vi "clickpoints.vi"(8 "Err_In":errorcluster) -> (0 "error out":errorcluster caption="Err_Out", 2 "MouseMoves":cdb[](array[numeric]), 3 "Points":cdb[](array[numeric]))   [LabVIEW 2012]
doc: "This VI can be used for interactive point definition. If you click with the left mouse key, the purrent position of the mouse (in screen coordinates) is added to an array.\nIf you click with another mouse button, the interactive point definition will be finished.\n\nThe VI works almost like \"mausi.vi\". The difference here: The VI will be finished by a click with the middle or right mouse key."
uses:
  <vilib>/Utility/inputDevices.llb/mouseAcquire.vi
  <vilib>/Utility/inputDevices.llb/closeMouse.vi
panel:
  out "NoOfPTS":i32
  out "Movement":bool
  out "XY-Graph":cluster{dbl[], dbl[]}[](graph)
  out "button info":T1 caption="KeyInfo"
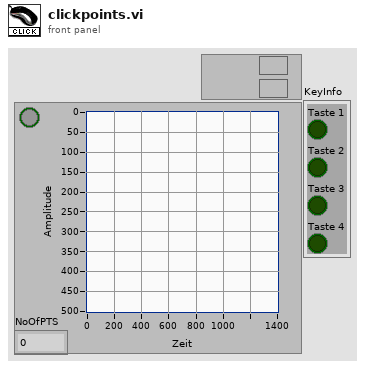
[diagram p1: front panel]
types:
  T1 = cluster{"button 1":bool, "button 2":bool, "button 3":bool, "button 4":bool}
  T2 = cluster{"Horizontal":i32, "Vertical":i32, "Scrolling":i32}
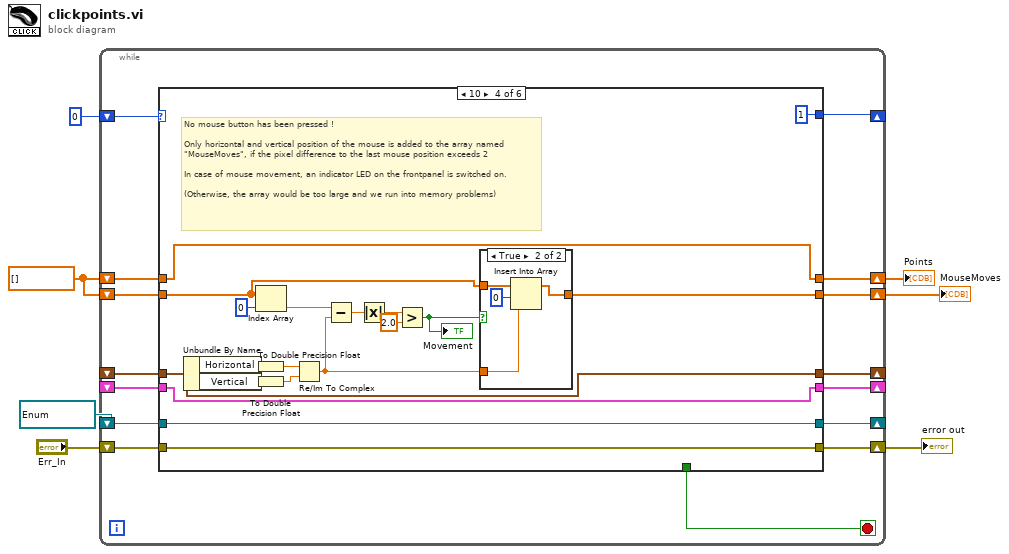
[diagram p0: block diagram]
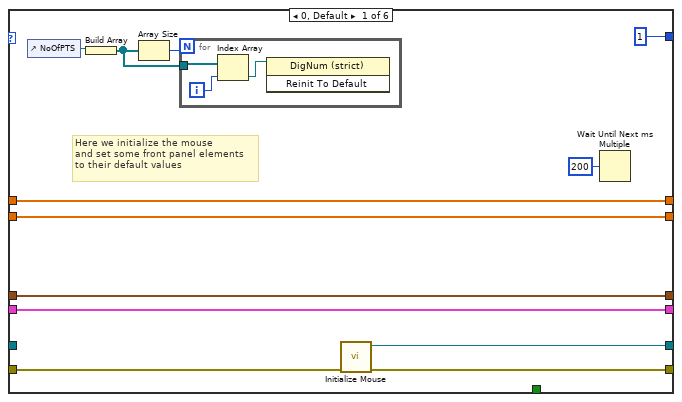
[diagram p2: hidden frame]
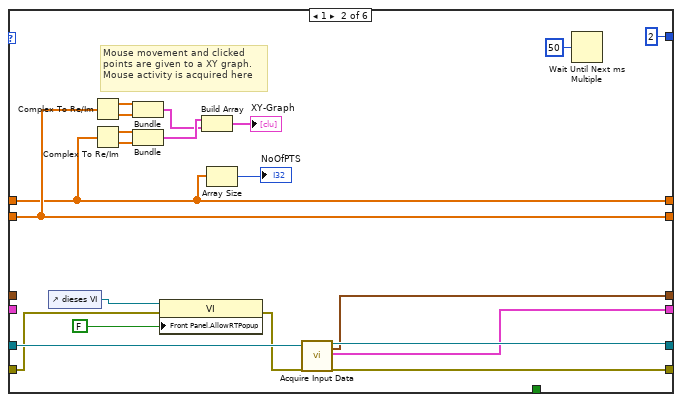
[diagram p3: hidden frame]
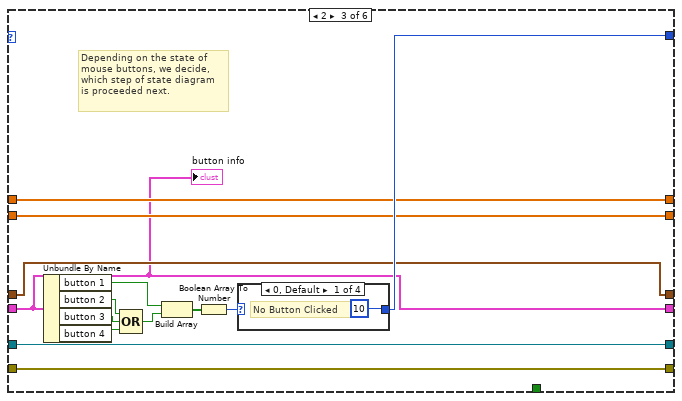
[diagram p4: hidden frame]
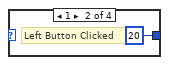
[diagram p5: hidden frame]
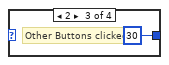
[diagram p6: hidden frame]
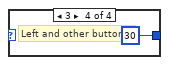
[diagram p7: hidden frame]
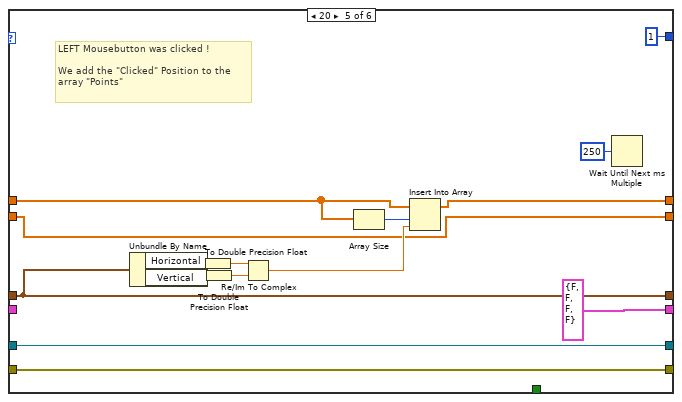
[diagram p9: hidden frame]
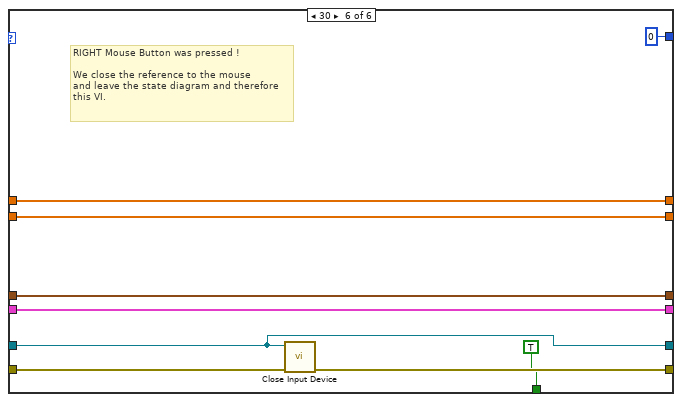
[diagram p10: hidden frame]
diagram:
  w1 = cdb[] []
  w4 = refnum<k1> refnum items=["MOUSE"] ("device ID")
  n1 = while {
    shift-right: [w20] -> w5
    shift-left: "Err_In" -> [w21]
    shift-right: [w19] -> _
    shift-left: w4 -> [w17]
    shift-right: [w18] -> _
    shift-left: 0 ("Numerisches Element") -> [w22]
    shift-right: [w16] -> _
    shift-left: _ -> [w13]
    shift-right: [w15] -> _
    shift-left: _ -> [w14]
    shift-right: [w12] -> w2
    shift-left: w1 -> [w11]
    shift-right: [w10] -> w3
    shift-left: w1 -> [w9]
    stop <- w8 stop-if-true
    n2 = case shown="10" w22 {
      tunnel: w21 -> [w34 w40 w60 w88 w104 w124]
      tunnel: [w33 w58 w60 w88 w104 w123] -> w20
      tunnel: [w32 w56 w61 w87 w105 w116] -> w19
      tunnel: [1 ("Numerisches Element") 2 ("Numerisches Element") w65 1 ("Numerisches Element") 1 ("Numerisches Element") 0 ("Numerisches Element")] -> w18
      tunnel: w17 -> [_ w57 w61 w87 w105 w116]
      tunnel: [w29 w54 w62 w85 w106 w121] -> w16
      tunnel: [w30 w53 w59 w86 T1 {"button 1"=FALSE, "button 2"=FALSE, "button 3"=FALSE, "button 4"=FALSE} ("button info") w122] -> w15
      tunnel: w14 -> [w30 _ w59 w86 _ w122]
      tunnel: w13 -> [w29 _ w62 w85 w106 w121]
      tunnel: [w27 w47 w64 w84 w109 w119] -> w12
      tunnel: w11 -> [w27 w47 w64 w91 w109 w119]
      tunnel: [w26 w45 w63 w89 w102 w118] -> w10
      tunnel: w9 -> [w26 w45 w63 w89 w103 w118]
      tunnel: [_ _ _ _ _ TRUE] -> w8
      frame 0, Default {
        # "Here we initialize the mouse\nand set some front panel elements\nto their default values"
        n3 = control-ref of="NoOfPTS"() -> (w23:refnum<vi>)
        n4 = Build Array(w23) -> (w24:refnum<vi>[])
        n5 = Array Size(array=w24) -> (size(s)=w25:i32)
        n6 = for {
          N: w25 -> [_]
          tunnel: w24 -> [w36]
          i -> [w37]
          n7 = Index Array(array=w36, index=w37) -> (element=w35:refnum<vi>)
          n8 = invoke class="DigNum (strict)" method="Reinit To Default"(reference=w35) -> ()  [unwired: 2 in, 3 out]
        }
        n9 = call <vilib>:"Initialize Mouse.vi"("error in (no error)"=w34) -> ("error out"=w33:errorcluster, "device ID"=w32:refnum<k1>)  [unwired: 9 out]
        n10 = Wait Until Next ms Multiple(millisecond multiple=u32 200 ("Vielfache von ms")) -> ()  [unwired: 1 out]
      }
      frame 1 {
        # "Mouse movement and clicked\npoints are given to a XY graph.\nMouse activity is acquired here"
        n11 = control-ref of="dieses VI"() -> (w41:refnum<vi>)
        n12 = Complex To Re/Im(x + iy=w47) -> (x=w51:dbl[], y=w50:dbl[])
        n13 = Complex To Re/Im(x + iy=w45) -> (x=w48:dbl[], y=w49:dbl[])
        n14 = Bundle(w51, w50) -> (w42:cluster{dbl[], dbl[]})  [unwired: 1 out]
        n15 = Bundle(w48, w49) -> (w43:cluster{dbl[], dbl[]})  [unwired: 1 out]
        n16 = property class="VI"(reference=w41, error in=w40, "Front Panel.AllowRTPopup"=FALSE ("Frontpanel-Fenster:Kontextmenü bei Ausführung möglich")) -> (error out=w39:errorcluster)  [unwired: 1 out]
        n17 = Build Array(w43, w42) -> (→"XY-Graph":cluster{dbl[], dbl[]}[])
        n18 = Array Size(array=w45) -> (size(s)=→"NoOfPTS":i32)
        n19 = call-poly <vilib>:"Acquire Input Data.vi"("device ID"=w57, "error in (no error)"=w39) -> ("device ID"=w56:refnum<k1>, "axis info"=w54:T2, "button info"=w53:T1, "error out"=w58:errorcluster)  [unwired: 1 in, 13 out]
        n20 = Wait Until Next ms Multiple(millisecond multiple=u32 50 ("Vielfache von ms")) -> ()  [unwired: 1 out]
      }
      frame 2 {
        # "Depending on the state of\nmouse buttons, we decide,\nwhich step of state diagram\nis proceeded next."
        n21 = Unbundle By Name(w59) -> ("button 1"=w69:bool, "button 2"=w70:bool, "button 3"=w71:bool, "button 4"=w72:bool)
        n22 = Compound Arithmetic op=OR(w70, w71, w72) -> (w68:bool)
        n23 = Build Array(w69, w68) -> (w67:bool[])
        n24 = Boolean Array To Number(Boolean array=w67) -> (number=w66:u32)
        n25 = case shown="0, Default" w66 {
          tunnel: [10 ("Numerisches Element") 20 ("Numerisches Element") 30 ("Numerisches Element") 30 ("Numerisches Element")] -> w65
          frame 0, Default {
            # "No Button Clicked"
          }
          frame 1 {
            # "Left Button Clicked"
          }
          frame 2 {
            # "Other Buttons clicked"
          }
          frame 3 {
            # "Left and other button"
          }
        }
        "button info" <- w59
      }
      frame 10 {
        # "No mouse button has been pressed !\n\nOnly horizontal and vertical position of the mouse is added to the array named \"MouseMoves\", if the pixel difference to the last mouse position exceeds 2\n\nIn case of mouse movement, an indicator LED on the frontpanel is switched on.\n\n(Otherwise, the array would be too large and we run into memory problems)"
        n26 = Unbundle By Name(w85) -> ("Horizontal"=w95:i32, "Vertical"=w94:i32)
        n27 = Index Array(array=w91, index=0 ("Index")) -> (element=w80:cdb)
        n28 = To Double Precision Float(number=w95) -> (double precision float=w93:dbl)
        n29 = To Double Precision Float(number=w94) -> (double precision float=w92:dbl)
        n30 = Re/Im To Complex(1:w92, 2:w93) -> (0:w79:cdb)
        n31 = Subtract(x=w80, y=w79) -> (x-y=w83:cdb)
        n32 = Absolute Value(x=w83) -> (abs(x)=w82:dbl)
        n33 = Greater?(x=w82, y=2.0) -> (0:w78:bool)
        "Movement" <- w78
        n34 = case shown="True" w78 {
          tunnel: [w96 w100] -> w84
          tunnel: w79 -> [_ w99]
          tunnel: w91 -> [w96 w98]
          frame False {
          }
          frame True {
            n35 = Insert Into Array(array=w98, index=0 ("Index"), new element=w99) -> (w100:cdb[])
          }
        }
      }
      frame 20 {
        # "LEFT Mousebutton was clicked !\n\nWe add the \"Clicked\" Position to the\narray \"Points\""
        n36 = Unbundle By Name(w106) -> ("Horizontal"=w115:i32, "Vertical"=w114:i32)
        n37 = To Double Precision Float(number=w115) -> (double precision float=w112:dbl)
        n38 = To Double Precision Float(number=w114) -> (double precision float=w113:dbl)
        n39 = Re/Im To Complex(1:w113, 2:w112) -> (0:w111:cdb)
        n40 = Array Size(array=w103) -> (size(s)=w110:i32)
        n41 = Insert Into Array(array=w103, index=w110, new element=w111) -> (w102:cdb[])
        n42 = Wait Until Next ms Multiple(millisecond multiple=u32 250 ("Vielfache von ms")) -> ()  [unwired: 1 out]
      }
      frame 30 {
        # "RIGHT Mouse Button was pressed !\n\nWe close the reference to the mouse\nand leave the state diagram and therefore\nthis VI."
        n43 = call-poly <vilib>:"Close Input Device.vi"("error in (no error)"=w124, "device ID"=w116) -> ("error out"=w123:errorcluster)  [unwired: 8 out]
      }
    }
  }
  "error out" <- w5
  "Points" <- w3
  "MouseMoves" <- w2
